vi "Highlight Golden Template Defects.vi"(7 "Defect Display Options":T1={"Show Bright Defects"=TRUE, "Bright Color"=6618880, "Show Dark Defects"=TRUE, "Dark Color"=16711680}, 8 "error in (no error)":errorcluster, 9 "Defect Image":T2, 10 "Destination Image":T2, 11 "Source Image":T2) -> (0 "error out":errorcluster, 2 "User Defined Color Palette":cluster{"Red":u8, "Green":u8, "Blue":u8}[](array[cluster]), 3 "Image Out":T2)   [LabVIEW 2016]
doc: "Modifies the source image to make it easy to display the results of the golden template comparison on the original image. The original image is adjusted so no pixels have a value less than 3. The Defect image is combined with this updated image so dark defects have a pixel value of 1, and bright defects have a pixel value of 2. A user defined color palette is output that has greyscale values for all pixel values except 1 (green by default) and 2 (red by default). To see these defects displayed, make sure to use a user defined palette for the image display and set the color palette to the User Defined Color Palette output by this VI."
uses:
  <vilib>/vision/Image Controls.llb/IMAQ Image.ctl
  <vilib>/vision/NI_Vision_Development_Module.lvlib
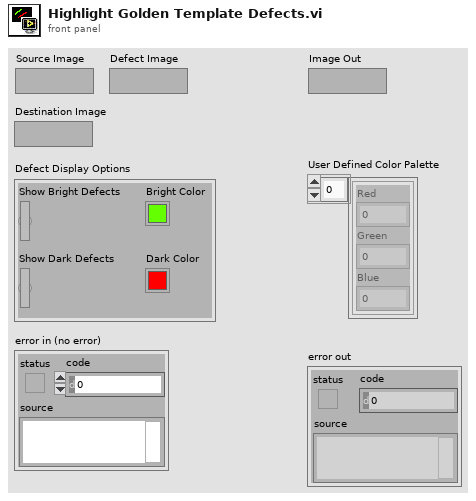
[diagram p1: front panel]
types:
  T1 = cluster{"Show Bright Defects":bool, "Bright Color":u32, "Show Dark Defects":bool, "Dark Color":u32}
  T2 = typedef "IMAQ Image.ctl" = refnum<image>
  T3 = enum32{"Gray", "Binary", "Gradient", "Rainbow", "Temperature"}
  T4 = cluster{"Red (or Hue) value":u8, "Green (or Sat) value":u8, "Blue (or Light or Val) value":u8}
  T5 = enum32{"Average", "Min", "Max", "Clear  if < ", "Clear  if < or =", "Clear  if =", "Clear  if > or =", "Clear  if >"}
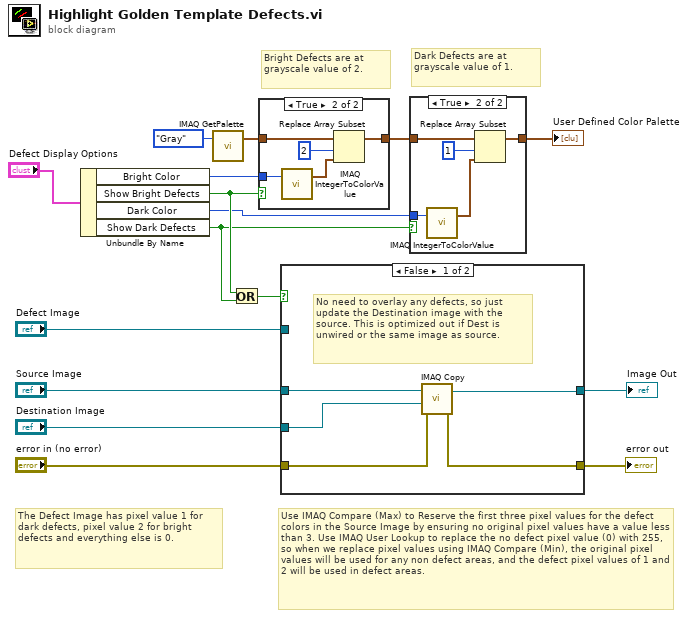
[diagram p0: block diagram]
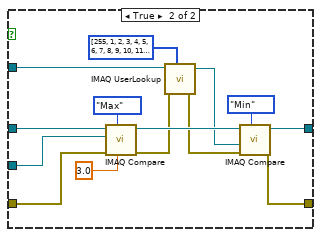
[diagram p2: hidden frame]
diagram:
  # "Use IMAQ Compare (Max) to Reserve the first three pixel values for the defect colors in the Source Image by ensuring no original pixel values have a value less than 3. Use IMAQ User Lookup to replace the no defect pixel value (0) with 255, so when we replace pixel values using IMAQ Compare (Min), the original pixel values will be used for any non defect areas, and the defect pixel values of 1 and 2 will be used in defect areas."
  # "The Defect Image has pixel value 1 for dark defects, pixel value 2 for bright defects and everything else is 0."
  # "Dark Defects are at grayscale value of 1."
  # "Bright Defects are at grayscale value of 2."
  n1 = Unbundle By Name("Defect Display Options") -> ("Bright Color"=w5:u32, "Show Bright Defects"=w6:bool, "Dark Color"=w3:u32, "Show Dark Defects"=w4:bool)
  n2 = call "IMAQ GetPalette"("Palette Number (gray)"=T3."Gray") -> ("Color Palette"=w16:cluster{"Red":u8, "Green":u8, "Blue":u8}[])  [unwired: 2 in, 3 out]
  n3 = Or(x=w6, y=w4) -> (x .or. y?=w13:bool)
  n4 = case shown="True" w6 {
    tunnel: w16 -> [w17 w22]
    tunnel: [w17 w21] -> w9
    tunnel: w5 -> [_ w18]
    frame False {
    }
    frame True {
      n5 = call "IMAQ IntegerToColorValue"("U32 value"=w18) -> ("Color Value"=w19:T4)  [unwired: 4 in, 3 out]
      n6 = Replace Array Subset(array=w22, new element=w19, index=2) -> (w21:cluster{"Red":u8, "Green":u8, "Blue":u8}[])
    }
  }
  n7 = case shown="False" w13 {
    tunnel: "Source Image" -> [w27 w35]
    tunnel: "Defect Image" -> [_ w34]
    tunnel: [w26 w36] -> w12
    tunnel: "Destination Image" -> [w25 w32]
    tunnel: "error in (no error)" -> [w24 w31]
    tunnel: [w23 w28] -> w1
    frame False {
      # "No need to overlay any defects, so just update the Destination image with the source. This is optimized out if Dest is unwired or the same image as source."
      n8 = call "IMAQ Copy"("error in (no error)"=w24, "Image Dst"=w25, "Image Src"=w27) -> ("error out"=w23:errorcluster, "Image Dst Out"=w26:T2)  [unwired: 3 in]
    }
    frame True {
      n9 = call "IMAQ Compare"("Constant"=sgl 3.0, "Operator"=T5."Max", "error in (no error)"=w31, "Image Dst"=w32, "Image Src A"=w35) -> ("error out"=w30:errorcluster, "Image Dst Out"=w40:T2)  [unwired: 1 in, 4 out]
      n10 = call "IMAQ UserLookup"("Image Src"=w34, "Lookup Table"=i16[] [255, 1, 2, 3, 4, 5, 6, 7, 8, 9, 10, 11, 12, 13, 14, 15, 16, 17, 18, 19, 20, 21, 22, 23, 24, 25, 26, 27, 28, 29, 30, 31, 32, 33, 34, 35, 36, 37, 38, 39, 40, 41, 42, 43, 44, 45, 46, 47, 48, 49, 50, 51, 52, 53, 54, 55, 56, 57, 58, 59, 60, 61, 62, 63, 64, 65, 66, 67, 68, 69, 70, 71, 72, 73, 74, 75, 76, 77, 78, 79, 80, 81, 82, 83, 84, 85, 86, 87, 88, 89, 90, 91, 92, 93, 94, 95, 96, 97, 98, 99, 100, 101, 102, 103, 104, 105, 106, 107, 108, 109, 110, 111, 112, 113, 114, 115, 116, 117, 118, 119, 120, 121, 122, 123, 124, 125, 126, 127, 128, 129, 130, 131, 132, 133, 134, 135, 136, 137, 138, 139, 140, 141, 142, 143, 144, 145, 146, 147, 148, 149, 150, 151, 152, 153, 154, 155, 156, 157, 158, 159, 160, 161, 162, 163, 164, 165, 166, 167, 168, 169, 170, 171, 172, 173, 174, 175, 176, 177, 178, 179, 180, 181, 182, 183, 184, 185, 186, 187, 188, 189, 190, 191, 192, 193, 194, 195, 196, 197, 198, 199, 200, 201, 202, 203, 204, 205, 206, 207, 208, 209, 210, 211, 212, 213, 214, 215, 216, 217, 218, 219, 220, 221, 222, 223, 224, 225, 226, 227, 228, 229, 230, 231, 232, 233, 234, 235, 236, 237, 238, 239, 240, 241, 242, 243, 244, 245, 246, 247, 248, 249, 250, 251, 252, 253, 254, 255], "error in (no error)"=w30) -> ("Image Dst Out"=w39:T2, "error out"=w29:errorcluster)  [unwired: 2 in, 2 out]
      n11 = call "IMAQ Compare"("Operator"=T5."Min", "error in (no error)"=w29, "Image Src B"=w39, "Image Src A"=w40) -> ("error out"=w28:errorcluster, "Image Dst Out"=w36:T2)  [unwired: 2 in, 4 out]
    }
  }
  "Image Out" <- w12
  "error out" <- w1
  n12 = case shown="True" w4 {
    tunnel: w9 -> [w42 w46]
    tunnel: [w42 w45] -> w14
    tunnel: w3 -> [_ w43]
    frame False {
    }
    frame True {
      n13 = call "IMAQ IntegerToColorValue"("U32 value"=w43) -> ("Color Value"=w44:T4)  [unwired: 4 in, 3 out]
      n14 = Replace Array Subset(array=w46, new element=w44, index=1) -> (w45:cluster{"Red":u8, "Green":u8, "Blue":u8}[])
    }
  }
  "User Defined Color Palette" <- w14
